vi "UHR-Fleezers Control (host) - 11.9.vi"() -> ()   [LabVIEW 2014] (continued)
  # "Trap Display:"
  # "APD Display:"
  # "Trap Manipulation"
  # "Data Saving"
  # "DAQ"
  # "Bead Calibration"
  # "Tether screen"
  # "Bottom Pump (#1)"
  # "Central Sample Channels"
  # "Top Pump (#3)"
  # "Rate param is ul/h\nVolume param is ul"
  # "Chemyx Pump 2"
  # "Units: \n1 = ml/m\n2 = ml/h\n3 = ul/m\n4 = ul/h"
  # "X"
  # "Y"
  # "Oscillate Set 1 freq. (debugging)"
  # "BD 1"
  # "BD 2"
  # "AOD Raster Scan"
  # "Approx. trap separations"
  # "X"
  # "Y"
  # "FPGA\nreading"
  # "DMA\ntransfer"
  # "APD Gates"
  # "APD 2"
  # "APD 1"
  # "X"
  # "2D"
  # "Y"
  # "1D"
  # "Green Laser Interlacing"
  # "Green FB Measurement"
  # "Digital Gate"
  # "Current Analog Control"
  # "Total AI Rates (NOT rates/trap)"
  # "(Samples/trap x Trap Sets)"
  # "(Samples/channel x\n8 if averaging (8 channels)\n4 if no averaging)"
  # "Trap 1"
  # "Trap 2"
  # "Flour./Trap 3"
  # "External Video Window"
  # "MCL Position Debugging"
  # "Temporary Control Storage\n(these used to be somewhere else, still want to keep them)"
  # "Y"
  # "X"
  # "Trap Position Difference Limits"
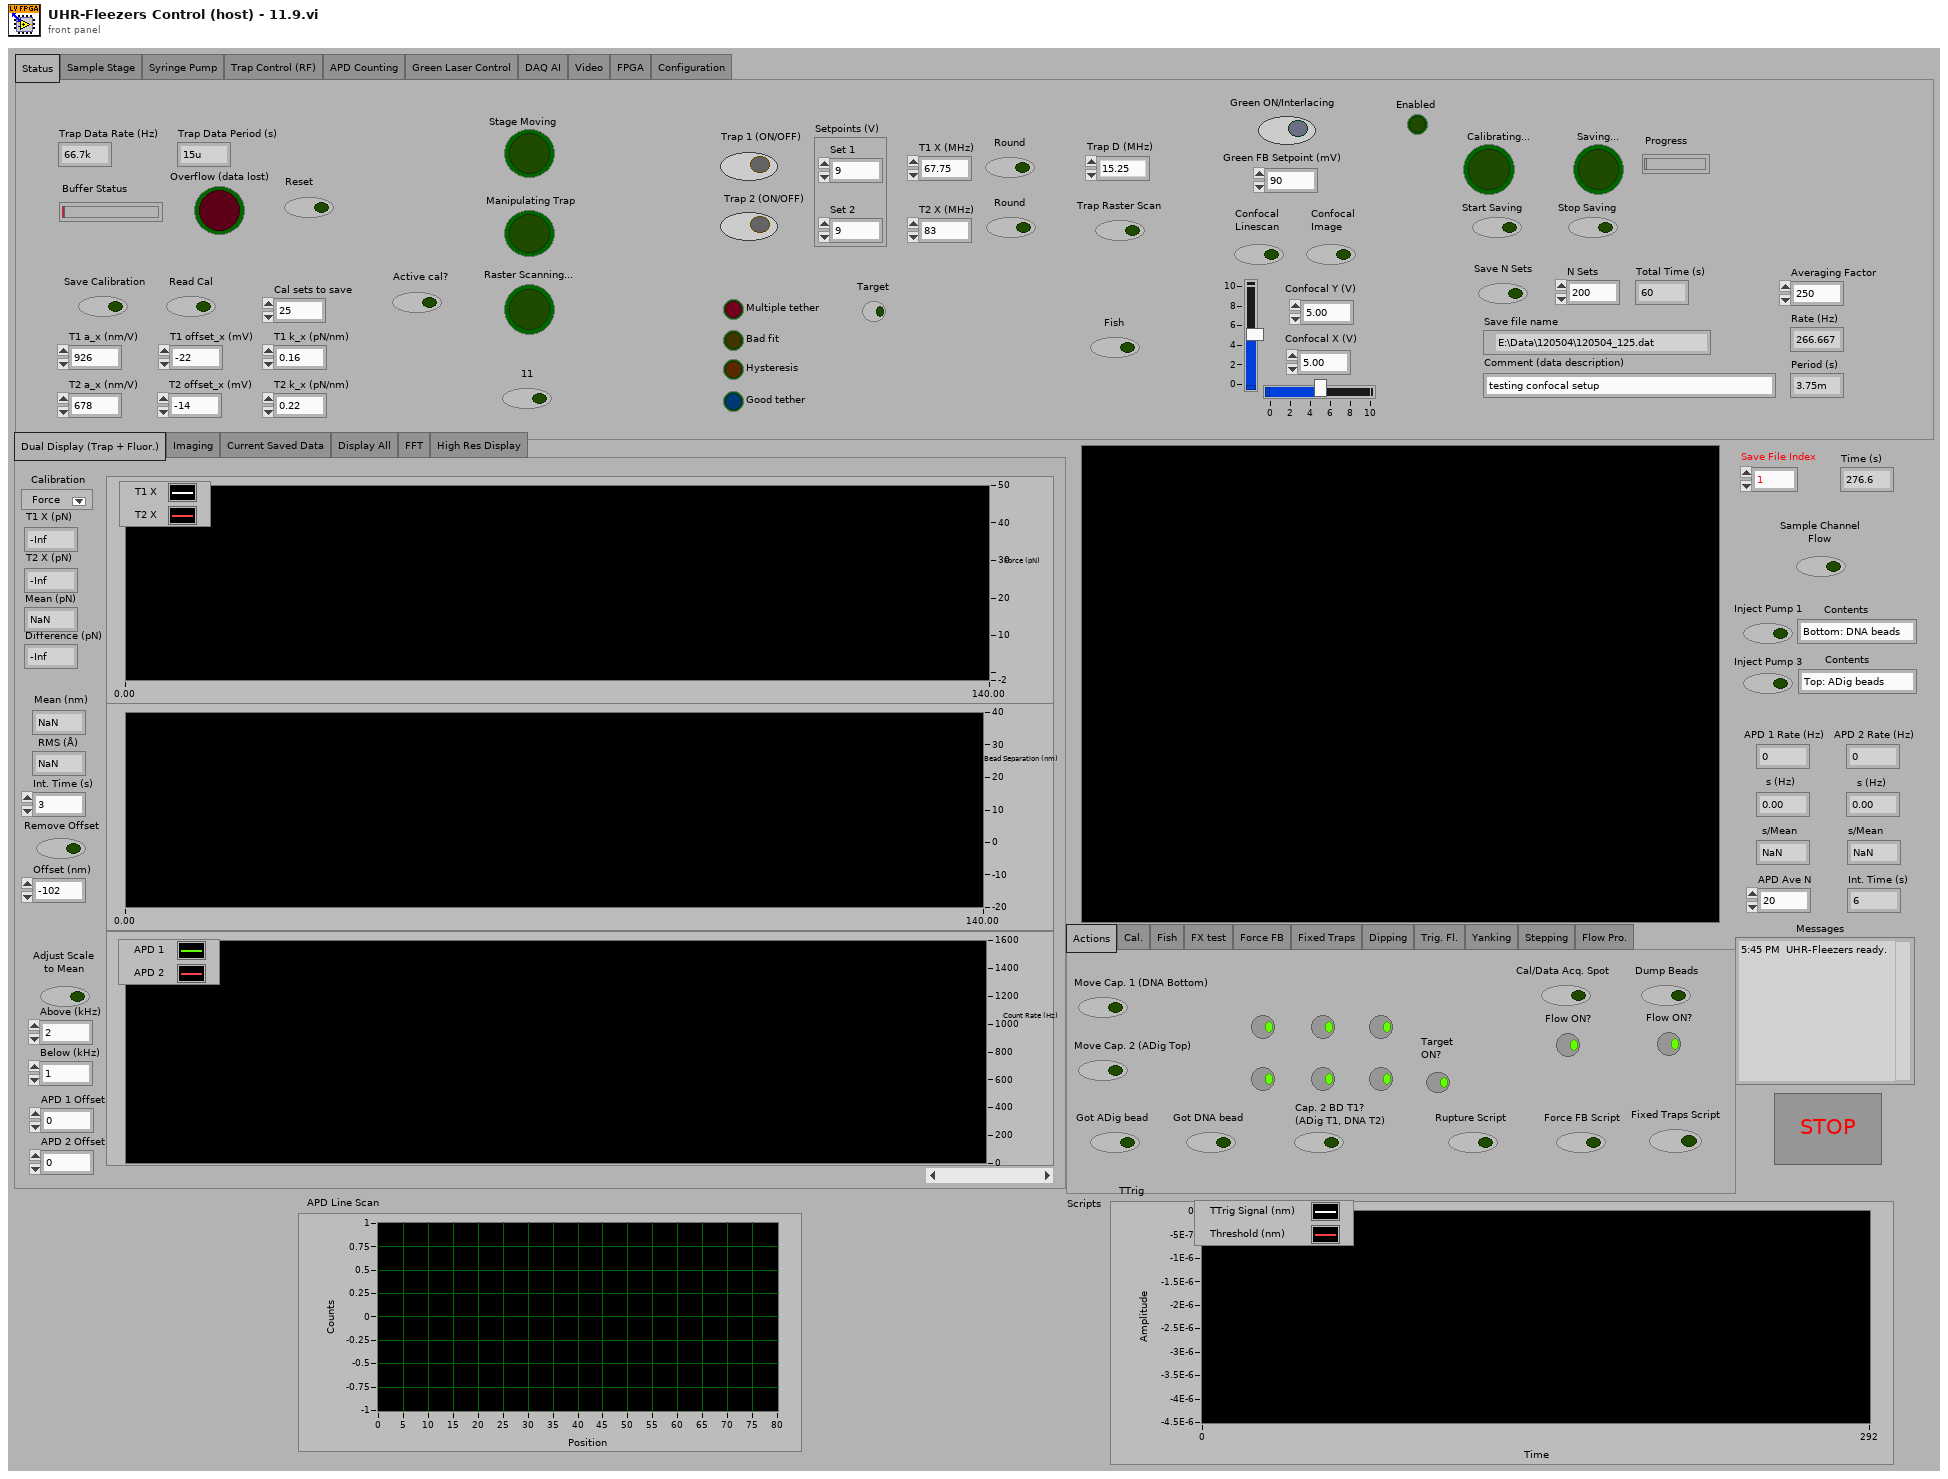
[diagram p1: front panel]
types:
  T1 = enum32{"Actions", "Cal.", "Fish", "FX test", "Force FB", "Fixed Traps", "Dipping", "Trig. Fl.", "Yanking", "Stepping", "Flow Pro."}
  T2 = typedef "IMAQ Image.ctl" = refnum<image>
  T3 = enum32{"Dual Display (Trap + Fluor.)", "Imaging", "Current Saved Data", "Display All", "FFT", "High Res Display"}
  T4 = enum32{"Status", "Sample Stage", "Syringe Pump", "Trap Control (RF)", "APD Counting", "Green Laser Control", "DAQ AI", "Video", "FPGA", "Configuration"}
  T5 = cluster{"Pump 1":cluster{"Diameter (mm)":dbl, "Units":dbl, "Volume":dbl, "Rate":dbl}, "Pump 2":cluster{"Diameter (mm)":dbl, "Units":dbl, "Volume":dbl, "Rate":dbl}, "Pump 3":cluster{"Diameter (mm)":dbl, "Units":dbl, "Volume":dbl, "Rate":dbl}}
  T6 = enum32{"IR Laser Interlacing (Direct RF Board Control Method)", "AOD Raster Scan", "Feedback on Trap Intensity", "Feedback on Trap Position"}
  T7 = typedef "LVPoint32TypeDef.ctl" = cluster{"Horizontal":i32, "Vertical":i32}
  T8 = cluster{"Scan Range AOD (nm) 2":dbl, "Step Size AOD (nm) 2":dbl, "Scan Speed AOD (nm/s) 2":dbl, "Number of scans (AOD) 2":u16, "Label":string}[]
  T9 = cluster{"Set 1":cluster{"proportional gain (Kc)":i16, "integral gain (Kc*Ts/Ti)":i16, "derivative gain (Kc*Td/Ts)":i16}, "Set 2":cluster{"proportional gain (Kc)":i16, "integral gain (Kc*Ts/Ti)":i16, "derivative gain (Kc*Td/Ts)":i16}}
  T10 = cluster{"Trap 1":fxp<+/-,16,1>, "Trap 2":fxp<+/-,16,1>}
  T11 = cluster{"proportional gain (Kc)":fxp<+/-,16,8>, "integral gain (Kc*Ts/Ti)":fxp<+/-,16,8>, "derivative gain (Kc*Td/Ts)":fxp<+/-,16,8>}
  T12 = cluster{"output high":fxp<+/-,64,32>, "output low":fxp<+/-,64,32>}
  T13 = cluster{"Set 1":fxp<+/-,16,1>, "Set 2":fxp<+/-,16,1>}
  T14 = cluster{"proportional gain (Kc)":i16, "integral gain (Kc*Ts/Ti)":i16, "derivative gain (Kc*Td/Ts)":i16}
  T15 = cluster{"Set 1":bool, "Set 2":bool, "Set 3":bool}
  T16 = typedef "LVMinMaxIncTypeDef.ctl" = cluster{"Minimum":dbl, "Maximum":dbl, "Increment":dbl}
  T17 = typedef "Image Type" = u32
  T18 = typedef "nirio_resource_hc.ctl" = tag
  T19 = typedef "openfpgaref.8.6.ctl" = refnum<k20>
  T20 = cluster{"New Image":T2, "New Image":T2, "New Image":T2, "New Image":T2}
  T21 = typedef "XDNodeRunTimeDep.lvlib/timing_clust.ctl" = cluster{"Expected End [f-1]":u64, "Actual End [f-1]":u64, "Finished Late? [f-1]":bool, "Expected End [i-1]":u64, "Actual End [i-1]":u64, "Finished Late? [i-1]":bool, "Expected Start [i]":u64, "Actual Start [i]":u64, "Expected Start [f]":u64, "Actual Start [f]":u64, "Source Name":string, "Structure Name":string, "Period":i64, "Deadline":i64, "Offset":i64, "Start":i64, "Priority":i32, "Timeout":i32, "Mode":T22, "Wakeup Reason":T23, "Error":errorcluster, "Source Type":string, "Secondary Source Type":string, "Global End Time":u64, "Global Start Time":u64, "Frame Duration":u64, "Iteration Duration":u64, "Assigned CPU":i32, "I/O Scan Engine Mode":u32}
  T22 = typedef "XDNodeRunTimeDep.lvlib/nitl_modes.ctl" = enum32{"No Change", "Process missed periods, maintain original phase", "Discard missed periods, maintain original phase", "Process missed periods, ignore original phase", "Discard missed periods, ignore original phase"}
  T23 = typedef "XDNodeRunTimeDep.lvlib/wakeup.ctl" = enum32{"Normal", "Aborted", "Asynchronous wakeup", "Timing source error", "Timed loop error", "Timeout"}
  T24 = enum16{"big-endian, network order", "native, host order", "little-endian"}
  T25 = enum16{"open", "replace", "create", "open or create", "replace or create", "replace or create with confirmation"}
  T26 = cluster{"Scan Range AOD (nm) 2":dbl, "Step Size AOD (nm) 2":dbl, "Scan Speed AOD (nm/s) 2":dbl, "Number of scans (AOD) 2":u16, "Label":string}
  T27 = cluster{"[0]":dbl, "[1]":dbl, "[2]":dbl, "[3]":dbl, "[4]":dbl, "[5]":dbl}
  T28 = cluster{"Diameter (mm)":dbl, "Units":dbl, "Volume":dbl, "Rate":dbl}
  T29 = enum16{"Actions", "Cal.", "Fish", "FX test", "Force FB", "Fixed Traps", "Dipping", "Trig. Fl.", "Yanking", "Stepping", "Flow Pro."}
  T30 = cluster{"Left":i32, "Top":i32, "Width":u32, "Height":u32}
  T31 = cluster{cluster{"Left":i32, "Top":i32, "Width":u32, "Height":u32}}[]
  T32 = enum32{"setting", "request", "request control", "info", "statistics", "system settings", "I/O sub system", "HRT control", "camera descriptions", "device specific data", "event sub system settings", "event sub system results", "image memory manager"}
  T33 = typedef "AviRefnum.ctl" = refnum<k1>
  T34 = typedef "imagedata.ctl" = cluster{"image type":i32, "image depth":i32, "image":u8[], "mask":u8[], "colors":u32[], "Rectangle":cluster{"left":i16, "top":i16, "right":i16, "bottom":i16}}
  T35 = enum32{"Normal Display", "Dual Display (APD)", "FFT", "High Res Display"}
  T36 = cluster{"Origin Pixel":cluster{"X":sgl, "Y":sgl}, "Angle Relative to Horizontal (deg)":sgl, "Axis Reference":u32}
  T37 = typedef "Simple Grid Descriptor" = cluster{"X Step":sgl, "Y Step":sgl, "Unit":T38}
  T38 = typedef "Image Unit" = enum32{"Undefined", "Angström", "Micrometer", "Millimeter", "Centimeter", "Meter", "Kilometer", "Microinch", "Inch", "Feet", "Nautical miles", "Standard miles", "Steps"}
  T39 = cluster{"averaging mode":u16, "weighting mode":u16, "number of averages":u32}
  T40 = cluster{"dB On (F)":bool, "unwrap phase (F)":bool, "convert to degree (F)":bool}
  T41 = cluster{string, string, string, string, string, string, string, string}
  T42 = cluster{string, string, string, string, string, string, string, string, string, string, string, string}
  T43 = cluster{string, string, string, string, string, string, string, string, string, string, string, string, string}
  T44 = cluster{string, string, string, string, string, string, string, string, string, string, string, string, string, string}
  T45 = cluster{"BD 1 Frequency 1 (MHz)":dbl, "BD 1 Frequency 2 (MHz)":dbl}
  T46 = cluster{"f0":dbl, "df":dbl, "magnitude":dbl[]}[][]
  T47 = cluster{"Green FB Ch 0":i16, "Green FB Ch 1":i16, "Green FB Ch 2":i16}
  T48 = cluster{"Green FB Ch 0":dbl, "Green FB Ch 1":dbl, "Green FB Ch 2":dbl}
diagram:
  w14 = 0.0 ("Total Volume\nFlowed P1 (uL)")
  w26 = u16 20 items=["1.0"=10, "1.5"=15, "2.0"=20] ("stop bits (10: 1 bit)")
  w29 = u16 20 items=["1.0"=10, "1.5"=15, "2.0"=20] ("stop bits (10: 1 bit)")
  w86 = u16 20 items=["1.0"=10, "1.5"=15, "2.0"=20] ("stop bits (10: 1 bit)")
  w93 = T17 2 items=["Grayscale (U8)", "Grayscale (I16)", "Grayscale (SGL)", "Complex (CSG)", "RGB (U32)", "HSL (U32)", "RGB (U64)", "Grayscale (U16)"] ("Image Type")
  w155 = cluster{"output high":i16, "output low":i16} {"output high"=3000, "output low"=0} ("FB output range 1")
  w226 = 10.0 ("y")
  w225 = 32767.0 ("y")
  w241 = 6.0  # clock mult.
  w242 = 49152000.0  # TCXO frequ.
  # "Bottom 1 Harvard"
  # "Top 3 Harvard"
  # "Center Harvard"
  # "Bottom 1 Harvard"
  # "Top 3 Harvard"
  # "Center Harvard"
  n1 = Build Array("DIO count 1 (ticks)", "DIO count 2 (ticks)", "DIO count 3 (ticks)") -> (w142:u32[])
  n2 = local read "AO1"() -> (w220:dbl)
  n3 = local read "AO2"() -> (w219:dbl)
  n4 = local read "Scan Increment (MHz)"() -> (w237:dbl)
  n5 = local read "Continuous MCL Scanning"() -> (w207:bool)
  n6 = local read "Fast Scan Dir"() -> (w206:bool)
  n7 = local read "Number of scans (MCL)"() -> (w208:u64)
  n8 = property on="AI Count (ticks)" class="DigNum (strict)"("Val(Sgnl)"="AI Count (ticks)") -> ()  [unwired: 2 in, 2 out]
  n9 = Multiply(x=w220, y=w225) -> (x*y=w222:dbl)
  n10 = Multiply(x=w219, y=w225) -> (x*y=w224:dbl)
  n11 = Divide(x=w222, y=w226) -> (x/y=w221:dbl)
  n12 = Divide(x=w224, y=w226) -> (x/y=w223:dbl)
  n13 = To Word Integer(number=w221) -> (16bit integer=w218:i16)
  n14 = To Word Integer(number=w223) -> (16bit integer=w217:i16)
  n15 = Not(x=w206) -> (.not. x?=w201:bool)
  n16 = local read "Cycles/step (MCL)"() -> (w209:u64)
  n17 = Multiply(x=w237, y=1000.0) -> (x*y=w244:dbl)
  n18 = local read "Scan steps (MCL)"() -> (w210:u64)
  n19 = local write "Trap Pos FIFO Timeout"(u16 0 ("Trap Pos FIFO Timeout")) -> ()
  n20 = local read "Desired Scan Incr (V)"() -> (w212:dbl)
  n21 = Scale By Power Of 2(n=48, x=w244) -> (x*2^n=w245:dbl)
  n22 = Multiply(x=w242, y=w241) -> (x*y=w240:dbl)
  n23 = Divide(x=w245, y=w240) -> (x/y=w239:dbl)
  n24 = local read "Setpoints (V)"() -> (w256:cluster{"Set 1":dbl, "Set 2":dbl})
  n25 = To Quad Integer(1:w239) -> (0:w236:i64)
  n26 = Divide(x=40000000.0, y="AI Count (ticks)") -> (x/y=w197:dbl)
  n27 = Multiply(x=w212, y=32767.0) -> (x*y=w214:dbl)
  n28 = local read "Number Interlace Sets"() -> (w135:u8)
  n29 = Split 1D Array(array=w142, index=w135) -> (first subarray=w144:u32[])  [unwired: 1 out]
  n30 = Add Array Elements(numeric array=w144) -> (sum=w143:u32)
  n31 = local read "# Samples/channel"() -> (w229:u32)
  n32 = local read "Number of F/B Scans (AOD)"() -> (w230:u16)
  n33 = local read "Not-Interlacing Set"() -> (w134:enum32{"Set 1", "Set 2", "Set 3"})
  n34 = To Unsigned Byte Integer(number=w134) -> (unsigned 8bit integer=w140:u8)
  n35 = Index Array(array=w142, index=w140) -> (element=w141:u32)
  n36 = local read "Feedback On/Off"() -> (w259:cluster{"Set 1":bool, "Set 2":bool})
  n37 = local read "PID Gains"() -> (w251:T9)
  n38 = local read "Scan steps (AOD)"() -> (w235:u64)
  n39 = local read "All FB On/Off"() -> (w260:bool)
  n40 = local read "Cycles/step (AOD)"() -> (w234:u64)
  n41 = local write "AI rate (Hz)"(w197) -> ()
  n42 = Divide(x=w214, y=10.0) -> (x/y=w213:dbl)
  n43 = Multiply(x=w235, y=w234) -> (x*y=w233:u64)
  n44 = Multiply(x=3276.7, y=w256) -> (x*y=w255:cluster{"Set 1":dbl, "Set 2":dbl})
  n45 = To Word Integer(number=w213) -> (16bit integer=w211:i16)
  n46 = xnode "Open FPGA VI Reference"("resource name"=T18 "RIO1") -> ("FPGA VI Reference Out"=w12:T19, "error out"=w10:errorcluster)  [unwired: 1 in]
  n47 = Multiply(x=w233, y=u64 2) -> (x*y=w231:u64)
  n48 = local read "Sets to FIFO (Traps)"() -> (w263:T15)
  n49 = Divide(x=w197, y="FPGA Ave.") -> (x/y=w198:dbl)
  n50 = To Word Integer(number=w255) -> (16bit integer=w254:cluster{"Set 1":i16, "Set 2":i16})
  n51 = Unbundle By Name(w251) -> ("Set 1"=w250:T14, "Set 2"=w249:T14)
  n52 = Multiply(x=w231, y=w230) -> (x*y=w228:u64)
  n53 = local write "Ave. Rate (Hz)"(w198) -> ()
  n54 = Divide(x=w228, y=w229) -> (x/y=w227:dbl)
  n55 = Unbundle By Name(w254) -> ("Set 1"=w253:i16, "Set 2"=w252:i16)
  n56 = local read "2D or 1D Scan"() -> (w156:bool)
  n57 = local write "Data points/scans"(w228) -> ()
  n58 = local read "Scan BD"() -> (w246:bool)
  n59 = And(x=w259, y=w260) -> (x .and. y?=w258:cluster{"Set 1":bool, "Set 2":bool})
  n60 = local write "Data points/scan (f/b)"(w231) -> ()
  n61 = Reciprocal(x=w198) -> (1/x=w199:dbl)
  n62 = local read "N Acq Sets (Traps + Fl.)"() -> (w190:i16)
  n63 = local write "N sets should be saved"(w227) -> ()
  n64 = xnode "Invoke Method"("FPGA VI Reference In"=w12, "error in"=w10) -> ("FPGA VI Reference Out"=w154:T19, "error out"=w164:errorcluster)
  n65 = Unbundle By Name(w258) -> ("Set 1"=w262:bool, "Set 2"=w261:bool)
  n66 = local read "Interlace"() -> (w136:bool)
  n67 = Select(t=w143, s=w136, f=w141) -> (s? t:f=w133:u32)
  n68 = local write "Update Count (MCL)"(w133) -> ()
  n69 = local write "Total Counts (ticks)"(w133) -> ()
  n70 = local write "Ave. Period (s)"(w199) -> ()
  n71 = property on="2D or 1D Scan" class="Bool (strict)"("Val(Sgnl)"=w156) -> ()  [unwired: 2 in, 2 out]
  n72 = local read "GI Frequency, OFF count"() -> (w58:u32)
  n73 = local read "GI Frequency, ON count"() -> (w49:u32)
  n74 = local read "APD Gate OFF Count"() -> (w55:u32)
  n75 = local read "APD Gate ON Count"() -> (w51:u32)
  n76 = xnode "Read/Write Control"("FPGA VI Reference In"=w153, "error in"=w164, "ai count"="AI Count (ticks)", "Interlace ON/OFF"=w136, "Number Interlace Cycles"=w135, "AI1 Sets to FIFO"=w263, "FB On/Off Set 1"=w262, "FB On/Off Set 2"=w261, "Interlace Off Parameters"=w134, "FB Setpoint Set 1"=w253, "FB Setpoint Set 2"=w252, "FB Gains Set 1"=w250, "FB Gains Set 2"=w249, "FB output range 1"=w155, "FB output range 2"=w155, "Cycles per step"=w234, "Scan BD"=w246, "Number of scans"=w230, "Scan steps"=w235, "Scan freq.  increment"=w236, "AO1"=w218, "AO2"=w217, "Scan freq.  increment (MCL)"=w211, "Scan steps (MCL)"=w210, "Cycles per step (MCL)"=w209, "Number of scans (MCL)"=w208, "MCL count"=w133, "Cont. Scan (MCL)"=w207, "MCL Scan Axis"=w201, "1D or 2D Scan?"=w156, "N of AI1 Int Acq Sets"=w190, "Freq or Amp switch first"="Freq or Amp switch first", "Freq switch delay"="Freq switch delay", "Amp switch delay"="Amp switch delay", "Swap F1 and F2"="Swap F1 and F2", "APD to FIFO"=FALSE, "DIO count 1 (ticks)"="DIO count 1 (ticks)", "DIO count 2 (ticks)"="DIO count 2 (ticks)", "DIO count 3 (ticks)"="DIO count 3 (ticks)") -> ("FPGA VI Reference Out"=w62:T19, "error out"=w60:errorcluster)  [unwired: 1 in]
  n77 = local read "On one out of X cycles"() -> (w57:u32)
  n78 = local read "APD Integration Time (s)"() -> (w41:dbl)
  n79 = local read "DMA Update Period (s)"() -> (w40:dbl)
  n80 = Add(x=w51, y=w55) -> (x+y=w53:u32)
  n81 = Add(x=w49, y=w58) -> (x+y=w56:u32)
  n82 = local read "Green ON/Interlacing"() -> (w131:bool)
  n83 = local read "Green laser mode"() -> (w132:enum32{"Laser ON", "Laser OFF", "Interlace"})
  n84 = Multiply(x=w53, y=w57) -> (x*y=w54:u32)
  n85 = Multiply(x=w57, y=w56) -> (x*y=w48:u32)
  n86 = Reciprocal(x=w41) -> (1/x=w38:dbl)
  n87 = Multiply(x=w41, y=40000000.0) -> (x*y=w37:dbl)
  n88 = Divide(x=w40, y=w41) -> (x/y=w43:dbl)
  n89 = Multiply(x="Current When FB OFF (%)", y=655.35) -> (x*y=w119:dbl)
  n90 = local read "Invert APD Gate"() -> (w47:bool)
  n91 = Multiply(x="Green FB Setpoint (mV)", y=3.2767) -> (x*y=w116:dbl)
  n92 = local read "APD Gate"() -> (w46:enum32{"ON", "OFF", "Interlace"})
  n93 = Subtract(x=w54, y=w51) -> (x-y=w52:u32)
  n94 = local write "Green FB Count"(w48) -> ()
  n95 = local write "APD Acq Rate (Hz)"(w38) -> ()
  n96 = To Unsigned Long Integer(number=w37) -> (unsigned 32bit integer=w35:u32)
  n97 = Multiply(x=2.0, y=w43) -> (x*y=w42:dbl)
  n98 = local read "Invert GI"() -> (w128:bool)
  n99 = To Unsigned Word Integer(number=w119) -> (unsigned 16bit integer=w117:u16)
  n100 = Subtract(x=w48, y=w49) -> (x-y=w50:u32)
  n101 = local write "APD Samples/FIFO Acq."(w43) -> ()
  n102 = To Word Integer(number=w116) -> (16bit integer=w114:i16)
  n103 = local write "APD Elements/DMA read"(w42) -> ()
  n104 = case shown="False" w131 {
    tunnel: w132 -> [_ w288]
    tunnel: [enum32{"Laser ON", "Laser OFF", "Interlace"}."Laser OFF" ("Green laser mode") w288] -> w127
    frame False {
    }
    frame True {
    }
  }
  n105 = local write "APD Int. Count"(w35) -> ()
  n106 = local read "Trap Pos. AI1 X Pre-scale"() -> (w72:u16)
  n107 = local read "Trap Pos FB Monitor\nT1 or T2"() -> (w79:bool)
  n108 = local read "Trap Pos FB Int Count"() -> (w66:u16)
  n109 = local read "APD 1 AO Mult."() -> (w45:i16)
  n110 = local read "Trap Pos FB Negate Action"() -> (w78:bool)
  n111 = local read "APD 2 AO Mult."() -> (w44:i16)
  n112 = local read "Trap Pos. FB Offset Factor"() -> (w77:i64)
  n113 = local read "Trap Pos. FB Mult Factor"() -> (w76:i64)
  n114 = local read "Differential FB?"() -> (w32:bool)
  n115 = local read "Neg. TTrig FPGA"() -> (w34:bool)
  n116 = local read "Trap Pos. FB Gains"() -> (w74:T11)
  n117 = local read "Trap Pos. FB Range"() -> (w75:T12)
  n118 = xnode "Read/Write Control"("FPGA VI Reference In"=w62, "error in"=w60, "Invert APD Gate"=w47, "APD Gate ON Count"=w51, "APD Gate OFF Count"=w52, "APD Acq Rate Count"=w35, "APD Gate Operating Mode"=w46, "APD 1 AO scale factor"=w45, "APD 2 AO scale factor"=w44, "Green interlace ON count"=w49, "Green interlace OFF count"=w50, "Green interlace ON count 2"=w49, "Green interlace OFF count 2"=w50, "Green FB Count"=w48) -> ("FPGA VI Reference Out"=w61:T19, "error out"=w59:errorcluster)
  n119 = xnode "Read/Write Control"("FPGA VI Reference In"=w61, "error in"=w59, "Invert GI 2"=w128, "Operating Mode 2"=w127, "Green FB Gains"="Green FB Gains", "Green FB Setpoint"=w114, "Green FB On/Off"="Green FB On/Off", "Current Out"=w117, "Green int current ON count adj"="Green int current ON count adj", "Operating Mode"=w127, "Invert GI"=w128, "Trap Pos FB Monitor T1 or T2"=w79, "Trap Pos FB Negate Action"=w78, "Trap Pos. FB Offset Factor"=w77, "Trap Pos. FB Mult Factor"=w76, "Trap Pos. FB Range"=w75, "Trap Pos. FB Gains"=w74, "Force feedback"=FALSE, "AI1 X Scale"=w72, "Trap Pos to FIFO"=TRUE, "Trap Pos FB Int Count"=w66, "TTrig Negate Pos"=w34, "FB Trig Integrate"="FB Trig Integrate", "Diff FB Measurement?"=w32, "Negate Diff?"="Negate Diff?") -> ("FPGA VI Reference Out"=w129:T19, "error out"=w130:errorcluster)
  n120 = xnode "Invoke Method"("FPGA VI Reference In"=w129, "error in"=w130, "Requested Depth"="Trap AI FIFO Depth") -> ("FPGA VI Reference Out"=w82:T19, "error out"=w81:errorcluster)  [unwired: 1 out]
  n121 = xnode "Invoke Method"("FPGA VI Reference In"=w82, "error in"=w81, "Requested Depth"="Trap Position FIFO Depth") -> ("FPGA VI Reference Out"=w68:T19, "error out"=w67:errorcluster)  [unwired: 1 out]
  n122 = flat-sequence {
    tunnel: w154 -> [w293]
    tunnel: [w293] -> w153
    tunnel: [w292] -> w152
    tunnel: [w291] -> w151
    tunnel: [w289] -> w149
    tunnel: [w290] -> w150
    frame #0 {
      w290 = T16 {"Minimum"=0.0, "Maximum"=40.0, "Increment"=1.0} ("Min Max Inc")
      w289 = T16 {"Minimum"=0.0, "Maximum"=50.0, "Increment"=1.0} ("Data Entry Limits")
      w292 = T16 {"Minimum"=60.0, "Maximum"=90.0, "Increment"=1.0} ("Min Max Inc")
      w291 = T16 {"Minimum"=0.0, "Maximum"=50.0, "Increment"=1.0} ("Data Entry Limits")
      n123 = property on="BD 2 Frequency 1 (MHz)" class="DigNum (strict)"("Data Range"=w290) -> ()  [unwired: 2 in, 2 out]
      n124 = property on="BD 2 Frequency 3 (MHz)" class="DigNum (strict)"("Data Range"=w290) -> ()  [unwired: 2 in, 2 out]
      n125 = property on="BD 2 Frequency 2 (MHz)" class="DigNum (strict)"("Data Range"=w290) -> ()  [unwired: 2 in, 2 out]
      n126 = property on="BD 1 Frequency 1 (MHz)" class="DigNum (strict)"("Data Range"=w292) -> ()  [unwired: 2 in, 2 out]
      n127 = property on="BD 1 Frequency 2 (MHz)" class="DigNum (strict)"("Data Range"=w292) -> ()  [unwired: 2 in, 2 out]
      n128 = property on="BD 1 Frequency 3 (MHz)" class="DigNum (strict)"("Data Range"=w292) -> ()  [unwired: 2 in, 2 out]
      n129 = property on="BD 2 Amplitude 1 (%)" class="DigNum (strict)"("Data Range"=w289) -> ()  [unwired: 2 in, 2 out]
      n130 = property on="BD 2 Amplitude 2 (%)" class="DigNum (strict)"("Data Range"=w289) -> ()  [unwired: 2 in, 2 out]
      n131 = property on="BD 2 Amplitude 3 (%)" class="DigNum (strict)"("Data Range"=w289) -> ()  [unwired: 2 in, 2 out]
      n132 = property on="BD 1 Amplitude 3 (%)" class="DigNum (strict)"("Data Range"=w291) -> ()  [unwired: 2 in, 2 out]
      n133 = property on="BD 1 Amplitude 2 (%)" class="DigNum (strict)"("Data Range"=w291) -> ()  [unwired: 2 in, 2 out]
      n134 = property on="BD 1 Amplitude 1 (%)" class="DigNum (strict)"("Data Range"=w291) -> ()  [unwired: 2 in, 2 out]
      "X RF Frequency Limits (MHz)" <- w292
      "X RF Amplitude Limits (%)" <- w291
      "Y RF Amplitude Limits (%)" <- w289
      "Y RF Frequency Limits (MHz)" <- w290
    }
  }
  n135 = xnode "Invoke Method"("FPGA VI Reference In"=w68, "error in"=w67) -> ("FPGA VI Reference Out"=w163:T19, "error out"=w162:errorcluster)  [unwired: 1 in]
  n136 = flat-sequence "Initial FPGA Loop Relative Phase Adjustment" {
    tunnel: "Initial Phase Adjustment (APD 2 Gate)" -> [w296]
    tunnel: "Initial Phase Adjustment (GI) 2" -> [w297]
    tunnel: "Initial Phase Adj. (MCL)" -> [w295]
    tunnel: w162 -> [w298]
    tunnel: w163 -> [w299]
    tunnel: "Initial Phase Adjustment (GI)" -> [w300]
    tunnel: "Initial Phase Adjustment (AI1)" -> [w301]
    tunnel: [w301] -> w9
    tunnel: [w300] -> w8
    tunnel: [w299] -> w7
    tunnel: [w298] -> w6
    tunnel: [w295] -> w5
    tunnel: [w297] -> w4
    tunnel: [w296] -> w3
    tunnel: [w313] -> w172
    tunnel: [w307] -> w168
    tunnel: "Initial Phase Adjustment (APD Acq)" -> [w306]
    tunnel: "Initial Phase Adjustment (APD 1 Gate)" -> [w305]
    tunnel: "Initial Phase Adjustment (Green FB)" -> [w304]
    tunnel: w9 -> [w312]
    tunnel: w8 -> [w311]
    tunnel: w7 -> [w310]
    tunnel: w6 -> [w309]
    tunnel: w5 -> [w308]
    tunnel: w4 -> [w303]
    tunnel: w3 -> [w302]
    tunnel: w172 -> [w315]
    tunnel: [w316] -> w169
    tunnel: w168 -> [w316]
    tunnel: [w315] -> w167
    tunnel: w169 -> [w319]
    tunnel: w167 -> [w318]
    tunnel: [w321] -> w166
    tunnel: [w320] -> w165
    tunnel: [w323] -> w170
    tunnel: [w324] -> w171
    tunnel: w166 -> [w324]
    tunnel: w165 -> [w323]
    frame #0 {
      n137 = Wait (ms)(milliseconds to wait=u32 100) -> ()  [unwired: 1 out]
    }
    frame #1 {
      n138 = xnode "Read/Write Control"("FPGA VI Reference In"=w310, "error in"=w309, "Phase count adjustment"=w312, "Phase count adjustment (GI)"=w311, "Phase count adjustment (MCL)"=w308, "Phase Count Adjustment (APD Acq)"=w306, "Phase count adjustment (APD 1 Gate)"=w305, "Phase count adjustment (APD 2 Gate)"=w302, "Phase count adjustment (Green FB)"=w304, "Phase count adjustment (GI) 2"=w303) -> ("FPGA VI Reference Out"=w307:T19, "error out"=w313:errorcluster)
    }
    frame #2 {
      n139 = Wait (ms)(milliseconds to wait=u32 100) -> ()  [unwired: 1 out]
    }
    frame #3 {
      w317 = TRUE
      n140 = xnode "Read/Write Control"("FPGA VI Reference In"=w319, "error in"=w318, "+ phase"=w317, "+ phase (GI)"=w317, "+ phase (MCL)"=w317, "+ phase (APD Acq)"=w317, "+ phase (APD 1 Gate)"=w317, "+ phase (APD 2 Gate)"=w317, "+ phase (Green FB)"=w317, "+ phase (GI) 2"=w317) -> ("FPGA VI Reference Out"=w320:T19, "error out"=w321:errorcluster)
    }
    frame #4 {
      n141 = Wait (ms)(milliseconds to wait=u32 100) -> ()  [unwired: 1 out]
    }
  }
  n142 = local read "Phase adj. (Green FB)"() -> (w145:i16)
  n143 = local read "Phase adj. (GI) 2"() -> (w120:i16)
  n144 = local read "Phase adjust (MCL)"() -> (w202:i16)
  n145 = local read "Phase adj. (AI1)"() -> (w204:i16)
  n146 = local read "Phase adj. (GI)"() -> (w203:i16)
  n147 = xnode "Read/Write Control"("FPGA VI Reference In"=w170, "error in"=w171, "Phase count adjustment"=w204, "Phase count adjustment (GI)"=w203, "Phase count adjustment (MCL)"=w202, "Phase Count Adjustment (APD Acq)"="Phase Adj. (APD Acq)", "Phase count adjustment (APD 1 Gate)"="Phase Adj. (APD 1 Gate)", "Phase count adjustment (APD 2 Gate)"="Phase Adj. (APD 2 Gate)", "Phase count adjustment (Green FB)"=w145, "Phase count adjustment (GI) 2"=w120) -> ("FPGA VI Reference Out"=w11:T19, "error out"=w179:errorcluster)
  n148 = call "Initialize RF boards - interlace 3.vi"("error in"=w179, "FPGA VI Reference In"=w11) -> ("error out"=w177:errorcluster, "FPGA VI Reference Out"=w178:T19)
  n149 = call "set RF board frequency - interlace.vi"("Board 2 Frequency Limits"=w150, "Board 1 Frequency Limits"=w152, "error in"=w177, "FPGA VI Reference In"=w178, "Board 2 Frequency 3 (MHz)"="BD 2 Frequency 3 (MHz)", "Board 1 Frequency 3 (MHz)"="BD 1 Frequency 3 (MHz)", "Board 2 Frequency 2 (MHz)"="BD 2 Frequency 2 (MHz)", "Board 2 Frequency 1 (MHz)"="BD 2 Frequency 1 (MHz)", "Board 1 Frequency 2 (MHz)"="BD 1 Frequency 2 (MHz)", "Board 1 Frequency 1  (MHz)"="BD 1 Frequency 1 (MHz)") -> ("error out"=w278:errorcluster, "FPGA VI Reference Out"=w279:T19)
  n150 = call "set RF board amplitude - interlace.vi"("Board 2 Amplitude Limits"=w149, "Board 1 Amplitude Limits"=w151, "error in"=w278, "FPGA VI Reference In"=w279, "Board 2 Amplitude 3 (%)"="BD 2 Amplitude 3 (%)", "Board 1 Amplitude 3 (%)"="BD 1 Amplitude 3 (%)", "Board 2 Amplitude 2 (%)"="BD 2 Amplitude 2 (%)", "Board 2 Amplitude 1 (%)"="BD 2 Amplitude 1 (%)", "Board 1 Amplitude 2 (%)"="BD 1 Amplitude 2 (%)", "Board 1 Amplitude 1 (%)"="BD 1 Amplitude 1 (%)") -> ("error out"=w266:errorcluster, "FPGA VI Reference Out"=w267:T19)
  n151 = flat-sequence {
    tunnel: w267 -> [w334]
    tunnel: w266 -> [w333]
    tunnel: [w332] -> w271
    tunnel: [w331] -> w270
    tunnel: [w338] -> w269
    tunnel: w271 -> [w338]
    tunnel: [w337] -> w268
    tunnel: w270 -> [w337]
    tunnel: w269 -> [w347]
    tunnel: w268 -> [w346]
    tunnel: [w345] -> w20
    tunnel: [w344] -> w69
    frame #0 {
      w325 = FALSE ("Retract Pump 3")
      n152 = local read "Trap 1 (ON/OFF)"() -> (w326:bool)
      n153 = xnode "Read/Write Control"("FPGA VI Reference In"=w334, "error in"=w333, "Direct RF Box  Communication"=FALSE) -> ("FPGA VI Reference Out"=w332:T19, "error out"=w331:errorcluster)
      n154 = local write "Saving..."(FALSE ("Saving Data")) -> ()
      n155 = local write "Stop All"(FALSE ("Stop All")) -> ()
      n156 = local write "Retract Pump 1"(w325) -> ()
      n157 = local write "Retract Pump 3"(w325) -> ()
      n158 = local write "Index"(1.0 ("Index")) -> ()
      n159 = property on="Trap 1 ON" class="Bool (strict)"("Value"=w326) -> ()  [unwired: 2 in, 2 out]
      "Manipulating Trap" <- FALSE ("Manipulating Trap")
    }
    frame #1 {
      n160 = local read "Trap 2 (ON/OFF)"() -> (w336:bool)
      n161 = Wait (ms)(milliseconds to wait=u32 10) -> ()  [unwired: 1 out]
      n162 = property on="Trap 2 ON" class="Bool (strict)"("Val(Sgnl)"=w336) -> ()  [unwired: 2 in, 2 out]
    }
    frame #2 {
      n163 = local read "Scan Range (nm)"() -> (w340:dbl)
      n164 = xnode "Read/Write Control"("FPGA VI Reference In"=w347, "error in"=w346, "FPGA Controls  RF Box"=TRUE ("Direct RF Box  Communication")) -> ("FPGA VI Reference Out"=w345:T19, "error out"=w344:errorcluster)
      n165 = call "Update messages.vi"("Message to add"="UHR-Fleezers ready.", "Old message string"="") -> ("New message string"=w343:string)
      n166 = local write "Messages"(w343) -> ()
      n167 = property on="Scan Range (nm)" class="DigNum (strict)"("Val(Sgnl)"=w340) -> ()  [unwired: 2 in, 2 out]
    }
  }
  n168 = Subtract(x="BD 1 Frequency 1 (MHz)", y="BD 1 Frequency 2 (MHz)") -> (x-y=w189:dbl)
  n169 = Subtract(x="BD 2 Frequency 1 (MHz)", y="BD 2 Frequency 2 (MHz)") -> (x-y=w188:dbl)
  n170 = Square(x=w188) -> (x^2=w186:dbl)
  n171 = Square(x=w189) -> (x^2=w187:dbl)
  n172 = Add(x=w187, y=w186) -> (x+y=w185:dbl)
  n173 = Square Root(x=w185) -> (sqrt(x)=w184:dbl)
  n174 = local write "Trap D (MHz)"(w184) -> ()
  n175 = call "IMAQ Create"("Image Name"="APD 1 Image", "Image Type"=w93) -> ("New Image"=w92:T2)  [unwired: 3 in, 1 out]
  n176 = call "IMAQ Create"("Image Name"="APD 2 Image", "Image Type"=w93) -> ("New Image"=w91:T2)  [unwired: 3 in, 1 out]
  n177 = call "IMAQ Create"("Image Name"="Det. X Image", "Image Type"=w93) -> ("New Image"=w90:T2)  [unwired: 3 in, 1 out]
  n178 = call "IMAQ Create"("Image Name"="Det. Y Image", "Image Type"=w93) -> ("New Image"=w89:T2)  [unwired: 3 in, 1 out]
  n179 = Bundle("New Image"=w92, "New Image"=w91, "New Image"=w90, "New Image"=w89) -> (w88:T20)  [unwired: 1 in]
  n180 = call-poly "VISA Configure Serial Port"("VISA resource name"="Bottom  1 Harvard Syringe Pump Serial Port", "baud rate (9600)"=u32 115200, "stop bits (10: 1 bit)"=w26) -> ("VISA resource name out"=w22:refnum<visa-resource-name>, "error out"=w21:errorcluster)  [unwired: 4 in, 7 out]
  n181 = call-poly "VISA Configure Serial Port"("VISA resource name"="Top 3 Harvard Syringe Pump Serial Port", "baud rate (9600)"=u32 115200, "stop bits (10: 1 bit)"=w29) -> ("VISA resource name out"=w24:refnum<visa-resource-name>, "error out"=w23:errorcluster)  [unwired: 4 in, 7 out]
  n182 = call-poly "VISA Configure Serial Port"("VISA resource name"="Sample Chamber Stage Serial Port") -> ("VISA resource name out"=w102:refnum<visa-resource-name>, "error out"=w103:errorcluster)  [unwired: 5 in, 8 out]
  "Stage Control Serial Error" <- w103
  n183 = call-poly "VISA Configure Serial Port"("VISA resource name"="Center Harvard Syringe Pump Serial Port", "baud rate (9600)"=u32 115200, "stop bits (10: 1 bit)"=w86) -> ("VISA resource name out"=w83:refnum<visa-resource-name>, "error out"=w84:errorcluster)  [unwired: 4 in, 7 out]
  n184 = disable-structure shown="Disabled" {
    disable-tunnel: [w350 _] -> w248
    disable-tunnel: w20 -> [w349 _]
    frame Disabled {
      n185 = node-c288() -> (w352:T21)  [unwired: 4 out]
      n186 = timed-loop "Rough control of MCL mirror stage (debugging)" {
        tunnel: w349 -> [w355]
        tunnel: [w354] -> w350
        timing: w352 -> [_]
        timing-out: [_] -> w351
        stop <- w354 stop-if-true
        n187 = node-c288() -> ()  [unwired: 2 out]
        n188 = case shown="1" "MCL Mode" {
          tunnel: w355 -> [_ w358 w405]
          frame 0, Default {
          }
          frame 1 {
            n189 = node-c288() -> (w360:T21)  [unwired: 4 out]
            n190 = timed-loop "Oscillate MCL mirror" {
              timing: w360 -> [_]
              timing-out: [_] -> w359
              tunnel: w358 -> [w399]
              i -> [w398]
              stop <- w361 stop-if-true
              n191 = node-c288() -> (w397:i64)  [unwired: 1 out]
              n192 = Multiply(x="AO1", y=32767.0) -> (x*y=w393:dbl)
              n193 = Multiply(x="AO2", y=32767.0) -> (x*y=w388:dbl)
              n194 = Divide(x=w393, y=10.0) -> (x/y=w394:dbl)
              n195 = Divide(x=w388, y=10.0) -> (x/y=w389:dbl)
              n196 = To Word Integer(number=w394) -> (16bit integer=w386:i16)
              n197 = To Word Integer(number=w389) -> (16bit integer=w385:i16)
              n198 = Divide(x=w397, y=i64 1000) -> (x/y=w368:dbl)
              n199 = Multiply(x=w368, y=w398) -> (x*y=w379:dbl)
              n200 = Multiply(x="Osc. freq. (Hz) 2", y=6.283185307179586) -> (x*y=w380:dbl)
              n201 = Multiply(x=w380, y=w379) -> (x*y=w378:dbl)
              n202 = Sine(x=w378) -> (sin(x)=w377:dbl)
              n203 = Multiply(x=w377, y="Osc. amp. (V)") -> (x*y=w375:dbl)
              n204 = Add(x=w375, y="Osc. center (V)") -> (x+y=w373:dbl)
              n205 = Divide(x=w373, y=10.0) -> (x/y=w371:dbl)
              n206 = Multiply(x=w371, y=32767.0) -> (x*y=w366:dbl)
              n207 = Select(t=w366, s="Scan axis", f=w386) -> (s? t:f=w384:dbl)
              n208 = Select(t=w385, s="Scan axis", f=w366) -> (s? t:f=w383:dbl)
              n209 = local read "MCL Mode"() -> (w365:u16)
              n210 = Not Equal?(x=w365, y=u16 1) -> (x != y?=w362:bool)
              n211 = local read "Stop All"() -> (w363:bool)
              n212 = xnode "Read/Write Control"("FPGA VI Reference In"=w399, "AO1"=w384, "AO2"=w383) -> ()  [unwired: 1 in, 2 out]
              n213 = Compound Arithmetic op=OR(w363, w362) -> (w361:bool)
              n214 = node-c288() -> ()  [unwired: 2 out]
            }
            n215 = node-c288(w359) -> ()  [unwired: 1 out]
          }
          frame 2 {
            n216 = case shown="True" "Start Scan" {
              tunnel: w405 -> [_ w417]
              frame False {
              }
              frame True {
                n217 = Subtract(x="End (V)", y="Begin (V)") -> (x-y=w413:dbl)
                n218 = Decrement(x="N Points") -> (x-1=w412:dbl)
                n219 = Divide(x=w413, y=w412) -> (x/y=w410:dbl)
                n220 = for {
                  N: "N Points" -> [_]
                  tunnel: "Begin (V)" -> [w430]
                  tunnel: w417 -> [w422]
                  tunnel: [w421] -> w416 mode=indexing
                  tunnel: w410 -> [w420]
                  tunnel: [w418] -> w409 mode=indexing
                  i -> [w429]
                  n221 = Multiply(x=w420, y=w429) -> (x*y=w428:dbl)
                  n222 = Add(x=w430, y=w428) -> (x+y=w425:dbl)
                  n223 = local read "Scan axis"() -> (w419:bool)
                  n224 = local read "AO1"() -> (w427:dbl)
                  n225 = local read "AO2"() -> (w426:dbl)
                  n226 = Select(t=w425, s=w419, f=w427) -> (s? t:f=w424:dbl)
                  n227 = Select(t=w426, s=w419, f=w425) -> (s? t:f=w423:dbl)
                  n228 = flat-sequence {
                    tunnel: w424 -> [w434]
                    tunnel: w423 -> [w433]
                    tunnel: w422 -> [w431]
                    tunnel: [w444] -> w421
                    tunnel: [w443] -> w418
                    frame #0 {
                      w437 = 10.0 ("y")
                      w432 = 32767.0 ("y")
                      n229 = Multiply(x=w434, y=w432) -> (x*y=w440:dbl)
                      n230 = Multiply(x=w433, y=w432) -> (x*y=w438:dbl)
                      n231 = Divide(x=w440, y=w437) -> (x/y=w441:dbl)
                      n232 = Divide(x=w438, y=w437) -> (x/y=w439:dbl)
                      n233 = To Word Integer(number=w441) -> (16bit integer=w435:i16)
                      n234 = To Word Integer(number=w439) -> (16bit integer=w436:i16)
                      n235 = xnode "Read/Write Control"("FPGA VI Reference In"=w431, "AO1"=w435, "AO2"=w436) -> ()  [unwired: 1 in, 2 out]
                    }
                    frame #1 {
                      n236 = Wait (ms)(milliseconds to wait="DAQ Delay (ms)") -> ()  [unwired: 1 out]
                    }
                    frame #2 {
                      n237 = local read "Slow mean"() -> (w444:dbl)
                      n238 = local read "Sigma"() -> (w443:dbl)
                    }
                  }
                }
                n239 = Bundle("Begin (V)"="Begin (V)", w410, w416) -> (→"MCL Scan":cluster{"Begin (V)":dbl, dbl, dbl[]})  [unwired: 1 out]
                n240 = Bundle("Begin (V)"="Begin (V)", w410, w409) -> (→"MCL Scan 2":cluster{"Begin (V)":dbl, dbl, dbl[]})  [unwired: 1 out]
              }
            }
          }
        }
        n241 = local read "Stop All"() -> (w354:bool)
        n242 = node-c288() -> ()  [unwired: 2 out]
      }
      n243 = node-c288(w351) -> ()  [unwired: 1 out]
    }
    frame Enabled {
    }
  }
  n244 = node-c288(3 ("Processor")) -> (w108:T21)  [unwired: 3 out]
  n245 = timed-loop "Oscillate Trap/AOM (fishing, debugging)" {
    tunnel: w20 -> [w448]
    tunnel: [w447] -> w113
    timing: w108 -> [_]
    timing-out: [_] -> w107
    stop <- w447 stop-if-true
    n246 = node-c288() -> ()  [unwired: 2 out]
    n247 = event shown="[0] \"Oscillate Set 1\", \"Fish\": Value Change" {
      selector: _ -> [_ _ _]
      dyn-events: _ -> [_ _ _]
      timeout: _ -> [_ _ _]
      tunnel: w448 -> [w455 _ _]
      tunnel: [FALSE ("Stop All") _ w1140] -> w447
      event "Oscillate Set 1", "Fish": Value Change {
        n248 = event-data() -> ()  [unwired: 6 out]
        n249 = local read "Oscillate Set 1"() -> (w454:bool)
        n250 = Or(x=w454, y="Fish") -> (x .or. y?=w452:bool)
        n251 = case shown="True" w452 {
          tunnel: w455 -> [_ w458]
          tunnel: "Fish" -> [_ w456]
          frame False {
          }
          frame True {
            n252 = case shown="True" w456 {
              selector: w456 -> [w461 w462]
              tunnel: [w461 w462] -> w457
              frame False {
              }
              frame True {
                w463 = FALSE ("Tether")
                n253 = local write "Scan axis 2"(TRUE) -> ()
                n254 = local write "Tether"(w463) -> ()
                n255 = local write "Hysteresis"(w463) -> ()
                n256 = local write "Multiple tether"(w463) -> ()
                n257 = local write "Bad fit"(w463) -> ()
                n258 = local write "Good tether"(w463) -> ()
                n259 = property on="Trap D (MHz)" class="DigNum (strict)"("Val(Sgnl)"="Furthest D (MHz)") -> ()  [unwired: 2 in, 2 out]
                n260 = local read "Flow ON\nduring cal?"() -> (w464:bool)
                n261 = Or(x="Flow ON during \nfishing?", y=w464) -> (x .or. y?=w465:bool)
                n262 = Wait (ms)(milliseconds to wait=u32 500) -> ()  [unwired: 1 out]
                n263 = property on="Sample Channel\nFlow" class="Bool (strict)"("Val(Sgnl)"=w465) -> ()  [unwired: 2 in, 2 out]
              }
            }
            n264 = node-c288() -> (w460:T21)  [unwired: 4 out]
            n265 = timed-loop "Oscillate AOD" {
              timing: w460 -> [_]
              timing-out: [_] -> w459
              tunnel: w458 -> [w477]
              tunnel: w457 -> [w471]
              i -> [w479]
              stop <- w470 stop-if-true
              n266 = node-c288() -> (w478:i64)  [unwired: 1 out]
              n267 = flat-sequence {
                tunnel: w479 -> [w506]
                tunnel: w478 -> [w505]
                tunnel: w477 -> [w484]
                tunnel: w471 -> [w487]
                tunnel: [w487] -> w476
                tunnel: [w486] -> w475
                tunnel: [w483] -> w474
                tunnel: [w480] -> w472
                tunnel: w476 -> [w549]
                tunnel: w475 -> [w547]
                tunnel: w474 -> [w546]
                tunnel: [w545] -> w473
                tunnel: w472 -> [w544]
                tunnel: [w705] -> w470
                tunnel: w473 -> [w704]
                frame #0 {
                  n268 = Divide(x=w505, y=i64 1000) -> (x/y=w500:dbl)
                  n269 = Multiply(x=w500, y=w506) -> (x*y=w502:dbl)
                  n270 = local read "BD 1 Frequency 2 (MHz)"() -> (w485:dbl)
                  n271 = Multiply(x="Osc. freq. (Hz)", y=6.283185307179586) -> (x*y=w503:dbl)
                  n272 = Multiply(x=w503, y=w502) -> (x*y=w482:dbl)
                  n273 = local read "BD 1 Frequency 1 (MHz)"() -> (w490:dbl)
                  n274 = local read "BD 2 Frequency 1 (MHz)"() -> (w489:dbl)
                  n275 = case shown="True" w487 {
                    tunnel: w482 -> [w512 w517]
                    tunnel: w490 -> [_ w528]
                    tunnel: w485 -> [_ w529]
                    tunnel: [w509 w523] -> w488
                    tunnel: [FALSE w520] -> w483
                    tunnel: [0.0 w513] -> w480
                    frame False {
                      n276 = Sine(x=w512) -> (sin(x)=w510:dbl)
                      n277 = Multiply(x=w510, y="Osc. amp. (MHz)") -> (x*y=w509:dbl)
                    }
                    frame True {
                      n278 = Cosine(x=w517) -> (cos(x)=w532:dbl)
                      n279 = Subtract(x=w529, y=w528) -> (x-y=w527:dbl)
                      n280 = Decrement(x=w532) -> (x-1=w531:dbl)
                      n281 = Subtract(x=w527, y="Closest D (MHz)") -> (x-y=w524:dbl)
                      n282 = Divide(x=w531, y=-2.0) -> (x/y=w525:dbl)
                      n283 = Multiply(x=w525, y=w524) -> (x*y=w523:dbl)
                      n284 = local read "Vec Mean of T1 T2"() -> (w519:dbl[])
                      n285 = Greater?(x=w519, y="Stop F (pN)") -> (0:w521:bool[])
                      n286 = Or Array Elements(Boolean array=w521) -> (logical OR=w520:bool)
                      n287 = Divide(x=w517, y=6.283185307179586) -> (x/y=w516:dbl)
                      n288 = Round Toward +Infinity(x=w516) -> (ceil(x): smallest int >= x=w513:dbl)
                      "Attempts" <- w513
                      n289 = Greater?(x=w513, y="Attempt Limit") -> (0:w515:bool)
                      n290 = case shown="True" w515 {
                        frame False {
                        }
                        frame True {
                          n291 = local write "Fish"(FALSE ("Fish for Tether")) -> ()
                          n292 = local read "Messages"() -> (w534:string)
                          n293 = flat-sequence {
                            frame #0 {
                              n294 = call <vilib>:"Beep.vi"("use system alert? (T)"=FALSE, "duration (msec)"=u32 200, "frequency (Hz)"=u32 500) -> ()  [unwired: 9 out]
                            }
                            frame #1 {
                              n295 = Wait (ms)(milliseconds to wait=u32 100) -> ()  [unwired: 1 out]
                            }
                            frame #2 {
                              n296 = call <vilib>:"Beep.vi"("use system alert? (T)"=FALSE, "duration (msec)"=u32 200, "frequency (Hz)"=u32 500) -> ()  [unwired: 9 in]
                            }
                          }
                          n297 = call "Update messages.vi"("Message to add"="Tether fishing timeout." ("Messages"), "Old message string"=w534) -> ("New message string"=→"Messages":string)
                        }
                      }
                    }
                  }
                  n298 = Select(t=w490, s="Scan axis 2", f=w489) -> (s? t:f=w493:dbl)
                  n299 = Add(x=w488, y=w493) -> (x+y=w486:dbl)
                  n300 = Select(t=w486, s="Scan axis 2", f=w490) -> (s? t:f=w496:dbl)
                  n301 = Select(t=w489, s="Scan axis 2", f=w486) -> (s? t:f=w495:dbl)
                  n302 = local read "Y RF Frequency Limits (MHz)"() -> (w491:T16)
                  n303 = local read "X RF Frequency Limits (MHz)"() -> (w492:T16)
                  n304 = local read "BD 2 Frequency 2 (MHz)"() -> (w498:dbl)
                  n305 = local read "BD 2 Frequency 3 (MHz)"() -> (w497:dbl)
                  n306 = local read "BD 1 Frequency 3 (MHz)"() -> (w499:dbl)
                  n307 = call "set RF board frequency - interlace.vi"("Board 2 Frequency Limits"=w491, "Board 1 Frequency Limits"=w492, "FPGA VI Reference In"=w484, "Board 2 Frequency 3 (MHz)"=w497, "Board 1 Frequency 3 (MHz)"=w499, "Board 2 Frequency 2 (MHz)"=w498, "Board 2 Frequency 1 (MHz)"=w495, "Board 1 Frequency 2 (MHz)"=w485, "Board 1 Frequency 1  (MHz)"=w496) -> ()  [unwired: 1 in, 2 out]
                }
                frame #1 {
                  n308 = And(x=w549, y=w546) -> (x .and. y?=w548:bool)
                  n309 = case "Only if were fishing and now formed tether" shown="True" w548 {
                    tunnel: w547 -> [w551 w566]
